vi "24HP_Open serial port.vi"(8 "Baud rate (bps)":u32=115200, 10 "timeout (ms)":u32=10000, 11 "VISA resource name":refnum<visa-resource-name>) -> (0 "Error out":errorcluster, 3 "VISA resource name out":refnum<visa-resource-name>)   [LabVIEW 2022 SP3]
uses:
  <vilib>/Instr/_visa.llb/VISA Open Access Mode.ctl
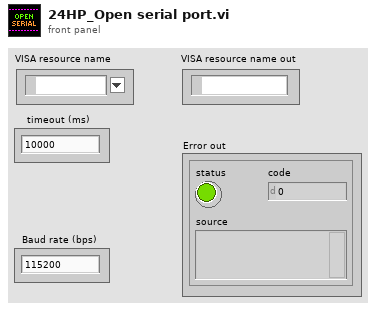
[diagram p1: front panel]
types:
  T1 = typedef "VISA Open Access Mode.ctl" = u32
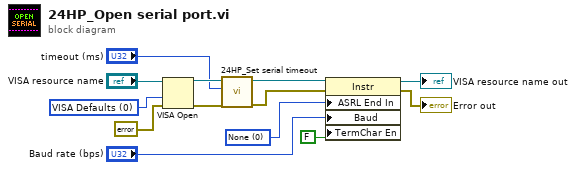
[diagram p0: block diagram]
diagram:
  w10 = u16 0 items=["None", "Last Bit", "TermChar"] ("Serial Settings:End Mode for Reads")
  w13 = T1 0 items=["VISA Defaults"=0, "Exclusive Lock"=1, "Load Configured Settings"=4] ("Access Mode")
  n1 = VISA Open(access mode=w13, error in (no error)=errorcluster {"status"=FALSE, "code"=0, "source"=""}, VISA resource name="VISA resource name") -> (VISA resource name=w6:refnum<visa-resource-name>, error out=w7:errorcluster)  [unwired: 2 in]
  n2 = call "24HP_Set serial timeout.vi"("Error In"=w7, "timeout (ms)"="timeout (ms)", "VISA resource name"=w6) -> ("Error Out"=w4:errorcluster, "VISA resource name out"=w5:refnum<visa-resource-name>)  [unwired: 7 in]
  n3 = property class="Instr"(reference=w5, error in=w4, "ASRL End In"=w10, "Baud"="Baud rate (bps)", "TermChar En"=FALSE ("Message Based Settings:Termination Character Enable")) -> (reference out=→"VISA resource name out":refnum<visa-resource-name>, error out=→"Error out":errorcluster)
